vi "Create Cal File Array (RIO).vi"() -> (0 "Cal Target Array":string[](array[string]), 3 "Cal Log OUT":string[][](array[string]))   [LabVIEW 2013]
uses:
  Type Defs/Units Type Def (DAQ Rack).ctl
  Type Defs/Channel Type Def (RIO).ctl
panel:
  in  "Channel to Cal":T1
  in  "Cal Unit":T2
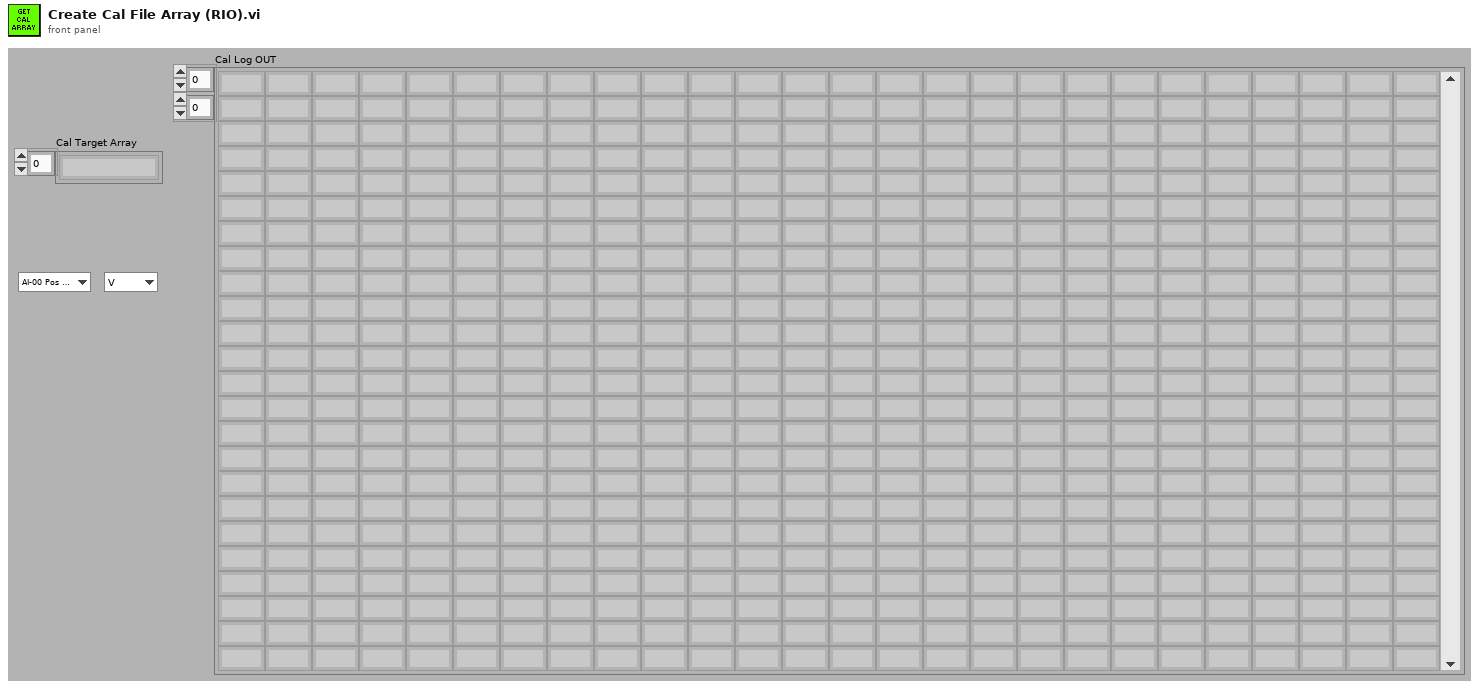
[diagram p1: front panel]
types:
  T1 = typedef "Channel Type Def (RIO).ctl" = enum16{"AI-00 Pos 1 Pump Current", "AI-01 Pos 2 Pump Current", "AI-02 Pos 3 Pump Current", "AI-03 Pos 4 Pump Current", "AI-04 Pos 5 Pump Current", "AI-05 Pos 6 Pump Current", "AI-06 Pos 1 Speed", "AI-07 Pos 2 speed", "AI-08 Pos 3 Speed", "AI-09 Pos 4 Speed", "AI-10 Pos 5 Speed", "AI-11 Pos 6 Speed", "AI-12 Pos 1 Controller Current", "AI-13 Pos 2 Controller Current", "AI-14 Pos 3 Controller Current", "AI-15 Pos 4 Controller Current", "AI-16 Pos 5 Controller Current", "AI-17 Pos 6 Controller Current", "AI-18 Spare", "AI-19 Tank 1 Temperature", "AI-20 Tank 2 Temperature", "AI-21 Power Supply Voltage", "AI-22 Pos 1 Pressure", "AI-23 Pos 2 Pressure", "AI-24 Pos 3 Pressure", "AI-25 Pos 4 Pressure", "AI-26 Pos 5 Pressure", "AI-27 Pos 6 Pressure", "AI-28 Pos 1 Flow", "AI-29 Pos 2 Flow", "AI-30 Pos 3 Flow", "AI-31 Pos 4 Flow", "AI-32 Pos 5 Flow", "AI-33 Pos 6 Flow", "AI-34 Spare", "AI-35 Spare", "AI-36 Spare", "AI-37 Spare"}
  T2 = typedef "Units Type Def (DAQ Rack).ctl" = enum16{"V", "mA", "A", "Hz", "deg C"}
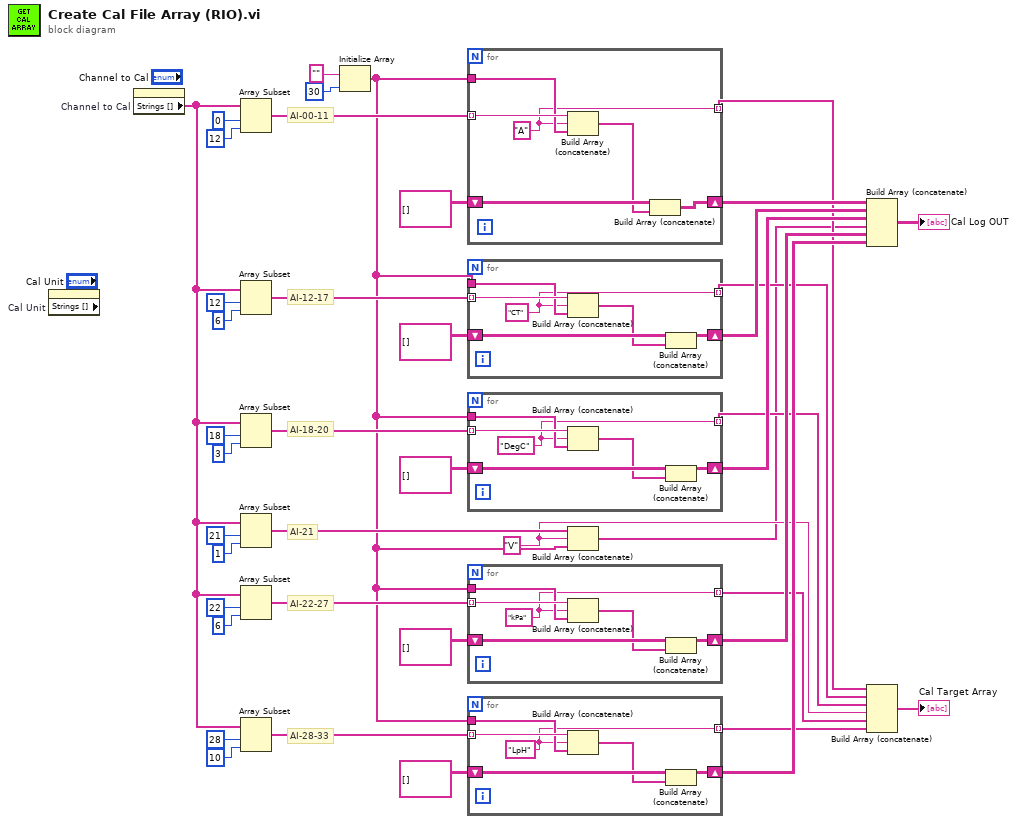
[diagram p0: block diagram]
diagram:
  w5 = "V"
  # "AI-28-33"
  # "AI-22-27"
  # "AI-21"
  # "AI-18-20"
  # "AI-12-17"
  # "AI-00-11"
  n1 = property on="Cal Unit" class="Enum (strict)" props=["Strings []"]() -> ()  [unwired: 2 in, 3 out]
  n2 = property on="Channel to Cal" class="Enum (strict)"() -> ("Strings []"=w20:string[])  [unwired: 2 in, 2 out]
  n3 = Array Subset(array=w20, index=0, length=12) -> (w37:string[])
  n4 = Array Subset(array=w20, index=12, length=6) -> (w32:string[])
  n5 = Array Subset(array=w20, index=18, length=3) -> (w13:string[])
  n6 = Array Subset(array=w20, index=21, length=1) -> (w14:string[])
  n7 = Array Subset(array=w20, index=22, length=6) -> (w15:string[])
  n8 = Array Subset(array=w20, index=28, length=10) -> (w16:string[])
  n9 = Initialize Array("", 30 ("dimension size")) -> (w12:string[])
  n10 = for {
    tunnel: w37 -> [w47] mode=indexing
    tunnel: w12 -> [w46]
    shift-right: [w44] -> w31
    shift-left: string[][] [] ("Cal Log OUT") -> [w45]
    tunnel: [w42] -> w2 mode=indexing
    w42 = "A"
    n11 = Build Array (concatenate)(w47, w42, w46) -> (w43:string[])
    n12 = Build Array (concatenate)(w45, w43) -> (w44:string[][])
  }
  n13 = for {
    tunnel: w32 -> [w51] mode=indexing
    tunnel: w12 -> [w49]
    shift-right: [w52] -> w29
    shift-left: string[][] [] ("Cal Log OUT") -> [w53]
    tunnel: [w48] -> w3 mode=indexing
    w48 = "CT"
    n14 = Build Array (concatenate)(w51, w48, w49) -> (w50:string[])
    n15 = Build Array (concatenate)(w53, w50) -> (w52:string[][])
  }
  n16 = for {
    tunnel: w13 -> [w57] mode=indexing
    tunnel: w12 -> [w55]
    shift-right: [w58] -> w11
    shift-left: string[][] [] ("Cal Log OUT") -> [w59]
    tunnel: [w54] -> w4 mode=indexing
    w54 = "DegC"
    n17 = Build Array (concatenate)(w57, w54, w55) -> (w56:string[])
    n18 = Build Array (concatenate)(w59, w56) -> (w58:string[][])
  }
  n19 = for {
    tunnel: w15 -> [w63] mode=indexing
    tunnel: w12 -> [w61]
    shift-right: [w64] -> w10
    shift-left: string[][] [] ("Cal Log OUT") -> [w65]
    tunnel: [w60] -> w6 mode=indexing
    w60 = "kPa"
    n20 = Build Array (concatenate)(w63, w60, w61) -> (w62:string[])
    n21 = Build Array (concatenate)(w65, w62) -> (w64:string[][])
  }
  n22 = for {
    tunnel: w16 -> [w69] mode=indexing
    tunnel: w12 -> [w67]
    shift-right: [w70] -> w9
    shift-left: string[][] [] ("Cal Log OUT") -> [w71]
    tunnel: [w66] -> w8 mode=indexing
    w66 = "LpH"
    n23 = Build Array (concatenate)(w69, w66, w67) -> (w68:string[])
    n24 = Build Array (concatenate)(w71, w68) -> (w70:string[][])
  }
  n25 = Build Array (concatenate)(w14, w5, w12) -> (w1:string[])
  n26 = Build Array (concatenate)(w31, w29, w11, w1, w10, w9) -> (→"Cal Log OUT":string[][])
  n27 = Build Array (concatenate)(w2, w3, w4, w5, w6, w8) -> (→"Cal Target Array":string[])
